vi "Cont Gen Current Updates Wfm-Int Clk.vi"() -> ()   [LabVIEW 2010]
doc: "I. Description:\nThis example demonstrates how to output a continuous number of current samples to an Analog Output Channel using an internal sample clock.\n\nII. Instructions for Running:\n1. Select the Physical Channel to correspond to where your signal is output on the DAQ device.\n2. Enter the Minimum and Maximum Current Ranges\n3. Specify the Desired Frequency of the output Waveform\n4. Enter the Waveform Information. See the documentation of the Waveform Buffer Generation SubVI for information on each parameter.\n\nIII. Block Diagram Steps:\n1. Create an Analog Output Current Channel.\n2. Call the DAQmx Timing (Use Waveform) VI which sets the sample clock rate based on the input waveform parameters, and set the sample mode to continuous.\n3. Use the Write VI to Generate Multiple Samples to 1 Channel on the Data Acquisition Card. The auto start parameter is set to False, so the Start VI must explicitly be called to begin the Current Generation. \n4. Call the Start VI.\n5. Call the Wait Until Done VI, with a time limit of 10s.\n6. Call the Clear Task VI to clear the Task.\n7. Use the popup dialog box to display an error or warning if any.\n\nIV. I/O Connections Overview:\nMake sure your signal output terminal matches the Physical Channel I/O Control. For further connection information, refer to your hardware reference manual."
uses:
  <vilib>/Utility/error.llb/DialogType.ctl
  <vilib>/DAQmx/write.llb/DAQmx Write (Analog 1D Wfm NChan NSamp).vi
  <vilib>/DAQmx/create/channels.llb/DAQmx Create Channel (AO-Current-Basic).vi
  <vilib>/DAQmx/configure/timing.llb/DAQmx Timing (Use Waveform).vi
  <vilib>/daqmx/miscellaneous.llb/DAQmx Fill In Error Info.vi
panel:
  in  "Offset":dbl=0.01 format="%0.2p"
  in  "Waveform Type":T1(ring)
  in  "stop":bool
  out "Resulting Frequency":dbl=1000.0 format="%.2f"
  in  "Cycles per Buffer":i32=5
  in  "Desired Frequency":dbl=1000.0 format="%.2f"
  in  "Samples per Buffer":dbl=250.0
  in  "Amplitude":dbl=0.01 format="%0.2p"
  in  "Minimum Value":dbl format="%0.2f"
  out "Output Waveform":waveform(dbl)[](graph)=[{"t0"=timestamp(0 s since 1904-01-01), "dt"=2e-05, "Y"=array[250 elements]}]
  in  "Maximum Value":dbl=0.02 format="%0.2f"
  in  "Physical Channel":tag="Dev1/ao0:1"
  # "For instructions, select Help>>Show Context Help"
  # "Channel Parameters"
  # "Timing Parameters"
  # "Waveform Information"
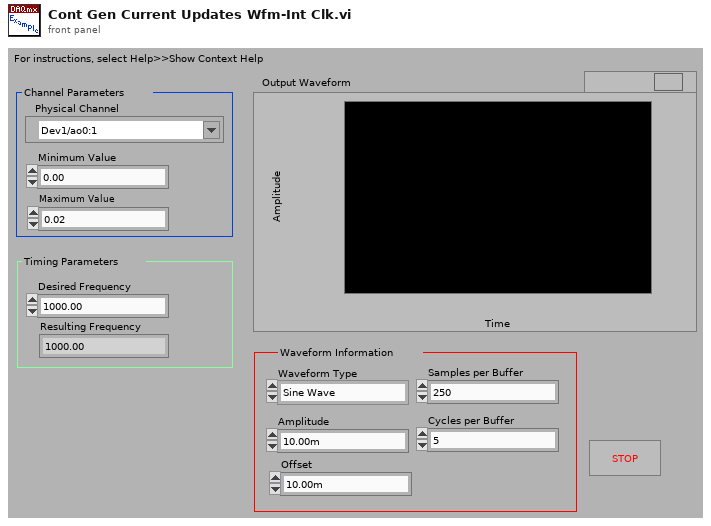
[diagram p1: front panel]
types:
  T1 = enum16{"Sine Wave", "Triangle Wave", "Square Wave", "Sawtooth Wave"}
  T2 = typedef "DialogType.ctl" = u16
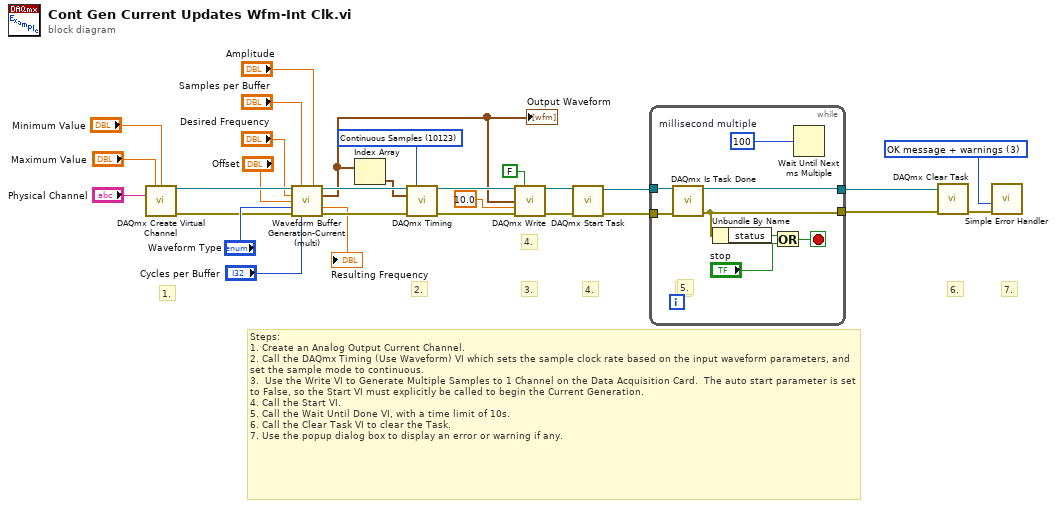
[diagram p0: block diagram]
diagram:
  w21 = 10123 items=["Finite Samples"=10178, "Continuous Samples"=10123] ("sample mode")
  w22 = T2 3 items=["no dialog", "OK message", "continue or stop message", "OK message + warnings", "continue/stop + warnings"] ("type of dialog (OK msg:1)")
  # "7."
  # "6."
  # "5."
  # "4."
  # "3."
  # "Steps: \n1. Create an Analog Output Current Channel.\n2. Call the DAQmx Timing (Use Waveform) VI which sets the sample clock rate based on the input waveform parameters, and set the sample mode to continuous.\n3.  Use the Write VI to Generate Multiple Samples to 1 Channel on the Data Acquisition Card.  The auto start parameter is set to False, so the Start VI must explicitly be called to begin the Current Generation.  \n4. Call the Start VI.\n5. Call the Wait Until Done VI, with a time limit of 10s.\n6. Call the Clear Task VI to clear the Task.\n7. Use the popup dialog box to display an error or warning if any."
  # "4."
  # "2."
  # "1."
  n1 = call-poly <vilib>:"DAQmx Create Virtual Channel.vi"("maximum value"="Maximum Value", "minimum value"="Minimum Value", "physical channels"="Physical Channel") -> ("task out"=w10:refnum<k21>, "error out"=w9:errorcluster)  [unwired: 11 in]
  n2 = call "Waveform Buffer Generation-Current (multi).vi"("task/channels in"=w10, "Samples per Buffer"="Samples per Buffer", "Amplitude"="Amplitude", "Desired Frequency"="Desired Frequency", "Offset"="Offset", "Waveform Type"="Waveform Type", "error in (no error)"=w9, "Cycles per Buffer"="Cycles per Buffer") -> ("task out"=w12:refnum<k21>, "Waveform"=w1:waveform(dbl)[], "Resulting Frequency"=→"Resulting Frequency":dbl, "error out"=w13:errorcluster)  [unwired: 3 in, 1 out]
  "Output Waveform" <- w1
  n3 = Index Array(array=w1) -> (element=w2:waveform(dbl))  [unwired: 1 in]
  n4 = call-poly <vilib>:"DAQmx Timing.vi"("task/channels in"=w12, "sample mode"=w21, "waveform"=w2, "error in"=w13) -> ("task out"=w28:refnum<k21>, "error out"=w27:errorcluster)  [unwired: 10 in]
  n5 = call-poly <vilib>:"DAQmx Write.vi"("task/channels in"=w28, "auto start"=FALSE, "data"=w1, "timeout"=10.0, "error in"=w27) -> ("task out"=w25:refnum<k21>, "error out"=w24:errorcluster)  [unwired: 8 in, 1 out]
  n6 = call <vilib>:"DAQmx Start Task.vi"("task/channels in"=w25, "error in"=w24) -> ("task out"=w18:refnum<k21>, "error out"=w17:errorcluster)  [unwired: 12 in]
  n7 = while {
    tunnel: w18 -> [w37]
    tunnel: [w36] -> w16
    tunnel: w17 -> [w35]
    tunnel: [w34] -> w15
    stop <- w32 stop-if-true
    w33 = u32 100  # millisecond multiple
    # "5."
    n8 = call <vilib>:"DAQmx Is Task Done.vi"("task/channels in"=w37, "error in"=w35) -> ("task out"=w36:refnum<k21>, "error out"=w34:errorcluster)  [unwired: 11 in, 1 out]
    n9 = Unbundle By Name(w34) -> ("status"=w31:bool)
    n10 = Or(x=w31, y="stop") -> (x .or. y?=w32:bool)
    n11 = Wait Until Next ms Multiple(millisecond multiple=w33) -> ()  [unwired: 1 out]
  }
  n12 = call <vilib>:"DAQmx Clear Task.vi"("task in"=w16, "error in"=w15) -> ("error out"=w23:errorcluster)  [unwired: 13 in]
  n13 = call <vilib>:"Simple Error Handler.vi"("type of dialog (OK msg:1)"=w22, "error in (no error)"=w23) -> ()  [unwired: 3 in, 5 out]
